vi "runTestScenario.vi"(0 "Digital Input Test  in":refnum<class "Verify ILC Test.lvclass">, 5 "ILC":refnum<class "ILC.lvclass">, 11 "error in (no error)":errorcluster) -> (4 "Digital Input Test out":refnum<class "Verify ILC Test.lvclass">, 6 "ILC 2":refnum<class "ILC.lvclass">, 8 "TestExecution":T2, 10 "Result":T1, 15 "error out":errorcluster)   [LabVIEW 2015, in "Verify ILC Test.lvclass"]
uses:
  Verify ILC Test.lvclass
  Typedefs/TestExecution.ctl
  Typedefs/PassFailTest.ctl
  <userlib>/Common/ILC/ILC/ILC.lvclass
  Typedefs/WriteLogMessageInput.ctl
  Typedefs/TestScenarioTypes.ctl
  Verify ILC Test.lvclass/Verify ILC Test.ctl
  Model/TestLog/ITestLog/ITestLog.lvclass
  Model/ConfigureILCStrategy/IConfigureILCStrategy/IConfigureILCStrategy.lvclass
  Model/ReadILCStrategy/IReadILCStrategy/IReadILCStrategy.lvclass
  Typedefs/ILCBTTypedefs.lvlib
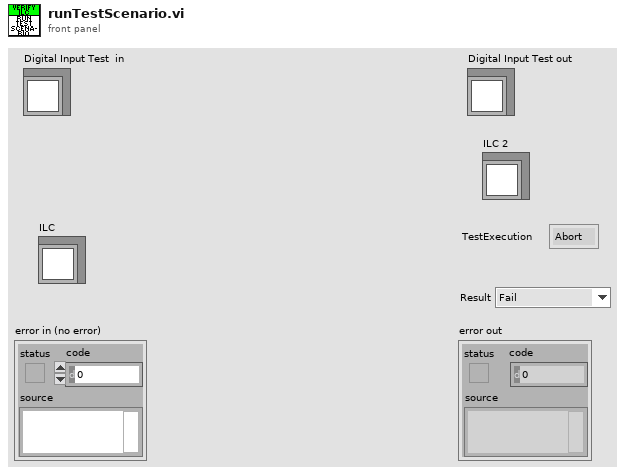
[diagram p1: front panel]
types:
  T1 = typedef "ILCBTTypedefs.lvlib/PassFailTest.ctl" = enum16{"Fail", "Pass", "NA"}
  T2 = typedef "ILCBTTypedefs.lvlib/TestExecution.ctl" = enum16{"Abort", "Continue"}
  T3 = typedef "ILCBTTypedefs.lvlib/WriteLogMessageInput.ctl" = cluster{"Test Scenario":T4, "Description":string, "Actual Value":string, "Data File":string, "Result":T1}
  T4 = typedef "ILCBTTypedefs.lvlib/TestScenarioTypes.ctl" = enum16{"+3.3VD", "+5.1V", "+24V", "RELVALV1", "RELVALV2", "Verify DAC_A = -1.00A", "Verify DAC_A = -0.75A", "Verify DAC_A = -0.50A", "Verify DAC_A = -0.25A", "Verify DAC_A = 0.00A", "Verify DAC_A = 0.25A", "Verify DAC_A = 0.50A", "Verify DAC_A = 0.75A", "Verify DAC_A = 1.00A", "Verify DAC_B = -1.00A", "Verify DAC_B = -0.75A", "Verify DAC_B = -0.50A", "Verify DAC_B = -0.25A", "Verify DAC_B = 0.00A", "Verify DAC_B = 0.25A", "Verify DAC_B = 0.50A", "Verify DAC_B = 0.75A", "Verify DAC_B = 1.00A", "Set DAC_A = -1.00A", "Set DAC_A = -0.75A", "Set DAC_A = -0.50A", "Set DAC_A = -0.25A", "Set DAC_A = 0.00A", "Set DAC_A = 0.25A", "Set DAC_A = 0.50A", "Set DAC_A = 0.75A", "Set DAC_A = 1.00A", "Set DAC_B = -1.00A", "Set DAC_B = -0.75A", "Set DAC_B = -0.50A", "Set DAC_B = -0.25A", "Set DAC_B = 0.00A", "Set DAC_B = 0.25A", "Set DAC_B = 0.50A", "Set DAC_B = 0.75A", "Set DAC_B = 1.00A", "Set MTR_PWR = On", "Set MTR_PWR = Off", "Set OUTPUT = On", "Set OUTPUT = Off"}
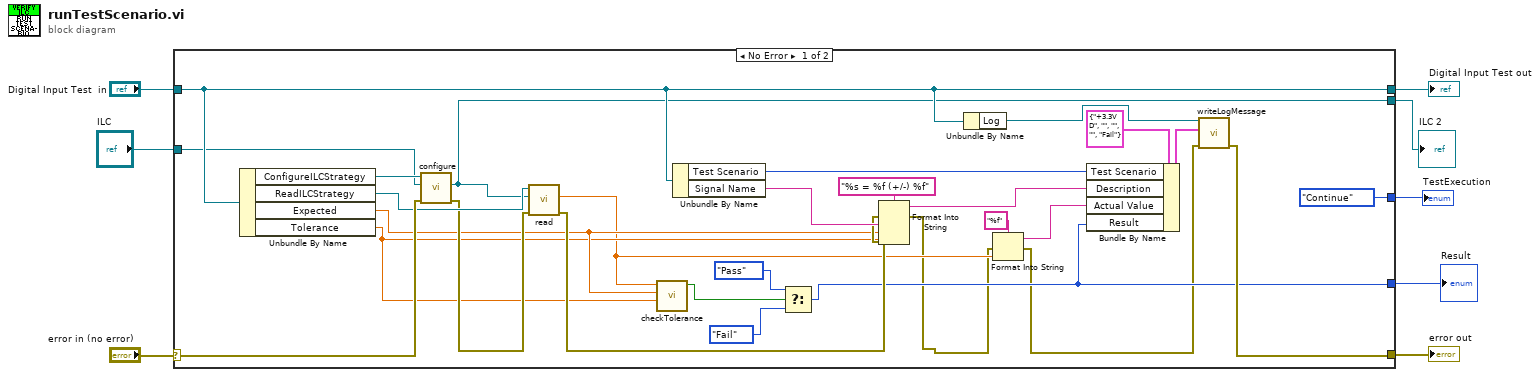
[diagram p0: block diagram]
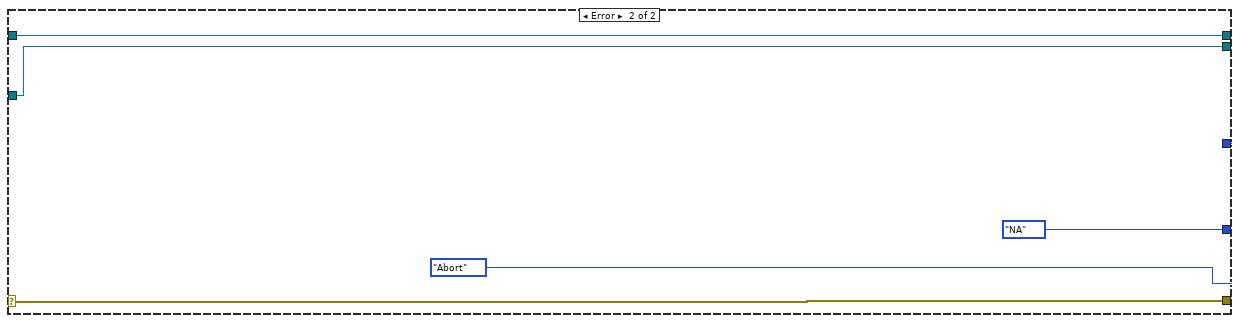
[diagram p2: hidden frame]
diagram:
  n1 = case shown="No Error" "error in (no error)" {
    selector: "error in (no error)" -> [w25 w41]
    tunnel: [w36 w41] -> w7
    tunnel: [TestExecution."Continue" ("TestExecution") TestExecution."Abort" ("TestExecution")] -> w6
    tunnel: "Digital Input Test  in" -> [w27 w39]
    tunnel: [w27 w39] -> w4
    tunnel: "ILC" -> [w24 w38]
    tunnel: [w14 PassFailTest."NA" ("Result")] -> w2
    tunnel: [w22 w38] -> w1
    frame No Error {
      n2 = Unbundle By Name(w27) -> ("ConfigureILCStrategy"=w34:refnum<class "IConfigureILCStrategy.lvclass">, "ReadILCStrategy"=w23:refnum<class "IReadILCStrategy.lvclass">, "Expected"=w19:dbl, "Tolerance"=w18:dbl)
      n3 = call-dynamic "configure.vi"("error in (no error)"=w25, "ILC"=w24, "IConfigureILCStrategy in"=w34) -> ("error out"=w21:errorcluster, "ILC 2"=w22:refnum<class "ILC.lvclass">)  [unwired: 6 in, 1 out]
      n4 = call-dynamic "read.vi"("error in (no error)"=w21, "ILC"=w22, "IReadILCStrategy in"=w23) -> ("error out"=w20:errorcluster, "Value"=w12:dbl)  [unwired: 6 in, 1 out]
      n5 = call "checkTolerance.vi"("Tolerance"=w18, "Expected Value"=w19, "Average"=w12) -> ("Boolean"=w17:bool)  [unwired: 8 in]
      n6 = Unbundle By Name(w27) -> ("Test Scenario"=w29:T4, "Signal Name"=w33:string)
      n7 = Select(t=PassFailTest."Pass" ("Result"), s=w17, f=PassFailTest."Fail" ("Result")) -> (s? t:f=w14:T1)
      n8 = Format Into String(format string="%s = %f (+/-) %f", error in=w20, w33, w19, w18) -> (resulting string=w30:string, error out=w10:errorcluster)  [unwired: 1 in]
      n9 = Unbundle By Name(w27) -> ("Log"=w26:refnum<class "ITestLog.lvclass">)
      n10 = Format Into String(format string="%f", error in=w10, w12) -> (resulting string=w11:string, error out=w9:errorcluster)  [unwired: 1 in]
      n11 = Bundle By Name(cluster=T3 {"Test Scenario"=enum."+3.3VD", "Description"="", "Actual Value"="", "Data File"="", "Result"=enum."Fail"} ("WriteLogMessageInput"), "Test Scenario"=w29, "Description"=w30, "Actual Value"=w11, "Result"=w14) -> (w31:T3)
      n12 = call-dynamic "writeLogMessage.vi"("error in (no error)"=w9, "WriteLogMessageInput"=w31, "ITestLog in"=w26) -> ("error out"=w36:errorcluster)  [unwired: 7 in, 1 out]
    }
    frame Error {
    }
  }
  "Digital Input Test out" <- w4
  "error out" <- w7
  "TestExecution" <- w6
  "Result" <- w2
  "ILC 2" <- w1
